vi "Mapping v10.6.3.2.vi"(5 "Simulate Spectra":bool, 7 "Simulate Drive":bool) -> ()   [LabVIEW 2010]
uses:
  TypeDefs/Mapping Spectra Params.ctl
  TypeDefs/Mapping Drive Params v10.6.0.ctl
  NPC3SG/TypeDefs/NPC3SG Set Positions.ctl
  NPC3SG/TypeDefs/NPC3SG Current Values.ctl
  iHR550/TypeDefs/iHR Current Values.ctl
  ITC503/TypeDefs/ITC503 Current Values.ctl
  TypeDefs/Mapping Input Parameters v10.6.2.ctl
  Symphony/TypeDefs/Symphony Area Format.ctl
  <vilib>/Utility/miscctls.llb/LVPointTypeDef.ctl
  Global Variables.vi
panel:
  in  "Measure Dummy 2":bool
  in  "Measure Dummy":bool
  in  "AutoSave Inc.":i16=20 caption="Auto Save (%)" min=10 max=160 step=1
  in  "Save Map":bool
  in  "Input Parameters":T1={"Drive Connection Port"="", "ITC503 Current Values"={"ITC503 Heater"=0.0, "ITC503 Temperature"=0.0, "ITC503 P"=0.0, "ITC503 I"=0.0, "ITC503 D"=0.0, "ITC503 Setpoint"=0.0, "ITC503 Gradient"=0.0, "ITC503 Heater Auto"=FALSE, "ITC503 PID Auto"=FALSE}, "Wavelengths (nm)"=[], "Drive Current Values"={"Drive X Position"=0.0, "Drive Y Position"=0.0, "Drive Z Position"=0.0}, "iHR Current Values"={"iHR 550 Front Entrance"=0.0, "iHR550 Side Exit"=0.0, "iHR550 Wavelength"=897.9988, "iHR550 Exit Mirror"=2, "iHR550 Grating"="1", "Grating Index"=1}, "Spectra Settings"={"Integration Time"=1.0, "Repetitions"=1, "Mapping Spectra"=TRUE}, "CCD3500 Temperature"=0.0, "Simulate Drive"=FALSE, "Simulate Spectra"=FALSE, "JYCCDLib.IJYCCDReqd"=refnum, "CCD Area"={"XStart"=1, "YStart"=1, "XStop"=2048, "YStop"=512, "XBin"=1, "YBin"=1}, "CCD Gain"=1, "CCD ADC"=0, "Drive Calibration"=path ""} {"CCD ADC" items=["20 kHz       ", " 1 MHz       ", " 1 MHz Ultra ", "500 kHz Wrap"]; "CCD Gain" items=["High Light", "Best Dynamic Range", "High Sensitivity"]; "ITC503 Current Values"."ITC503 Gradient" format="%.2f"; "ITC503 Current Values"."ITC503 Setpoint" min=-273.0 max=300000.0 step=0.0001 format="%.1f"; "ITC503 Current Values"."ITC503 I" format="%_1f"; "ITC503 Current Values"."ITC503 P" format="%_1f"; "ITC503 Current Values"."ITC503 Temperature" min=0.0 max=1645.0 step=1e-05 format="%.2f"; "ITC503 Current Values"."ITC503 Heater" min=0.0 max=100.0 step=0.01 scale=0.0..100.0; "Drive Current Values"."Drive Z Position" min=-273.0 max=300000.0 step=0.0001 format="%.3f"; "Drive Current Values"."Drive Y Position" min=-273.0 max=300000.0 step=0.0001 format="%.3f"; "Drive Current Values"."Drive X Position" min=-273.0 max=300000.0 step=0.0001 format="%.3f"; "iHR Current Values"."iHR550 Exit Mirror" items=["EntranceMirror", "ExitMirror", "Front", "Side"]; "Spectra Settings"."Repetitions" min=1 max=100 step=1; "Spectra Settings"."Integration Time" min=0.5 max=6000.0 step=1.0 format="%.1f"}
  out "JYCCDLib.IJYCCDReqd":refnum<k7>
  out "AutoClose":bool
  out "ITC503 Temperature":dbl caption="Sample (K)" min=10.0 max=160.0 step=0.1 format="%.3f"
  out "CCD3500 Temperature":dbl caption="CCD (°C)" min=10.0 max=160.0 step=0.1 format="%.1f"
  in  "CCD Current Rep.":string="0/0"
  in  "Pause":bool
  out "Current Position":T3 {"Drive Z Position" min=-273.0 max=300000.0 step=0.0001 format="%.3f"; "Drive Y Position" min=-273.0 max=300000.0 step=0.0001 format="%.3f"; "Drive X Position" min=-273.0 max=300000.0 step=0.0001 format="%.3f"}
  out "Target Position":T7={"Drive X Set"=10.0, "Drive Y Set"=10.0, "Drive Z Set"=10.0} {"Drive X Set" min=10.0 max=160.0 step=0.1 format="%.3f"; "Drive Z Set" min=10.0 max=160.0 step=0.1 format="%.3f"; "Drive Y Set" min=10.0 max=160.0 step=0.1 format="%.3f"}
  out "Progress":u8(slide) max=10 scale=0.0..100.0
  out "Objective Running":bool caption="Obj."
  out "CCD Running":bool caption="CCD"
  in  "Spectra Params":T5={"Integration Time"=10.0, "Repetitions"=10, "Mapping Spectra"=TRUE} {"Repetitions" min=1 max=100 step=1; "Integration Time" min=0.5 max=6000.0 step=1.0 format="%.1f"}
  in  "Drive Settings":refnum<visa-resource-name>
  in  "Z Position":dbl caption="Z (µm)" min=0.0 max=100.0 step=0.1 format="%.1f"
  in  "Mapping Params":T8={"X Start Position"=0.0, "X Stop Position"=10.0, "Y Start Position"=0.0, "Y Stop Position"=10.0, "Step Size"=1.0} {"Step Size" min=0.005 max=20.0 step=0.005 format="%.3f"; "Y Stop Position" min=0.0 max=140.0 step=0.005 format="%.3f"; "Y Start Position" min=0.0 max=140.0 step=0.005 format="%.3f"; "X Stop Position" min=0.0 max=140.0 step=0.005 format="%.3f"; "X Start Position" min=0.0 max=140.0 step=0.005 format="%.3f"}
  in  "Exit":bool
  out "Measuring":bool
  in  "Start":bool
  out "Filename":string
  out "Full Data":dbl[][](array[numeric])
  out "Live Data":dbl[][](array[numeric])
  in  "ITC503 Current Values":T2 {"ITC503 Gradient" format="%.2f"; "ITC503 Setpoint" min=-273.0 max=300000.0 step=0.0001 format="%.1f"; "ITC503 I" format="%_1f"; "ITC503 P" format="%_1f"; "ITC503 Temperature" min=0.0 max=1645.0 step=1e-05 format="%.2f"; "ITC503 Heater" min=0.0 max=100.0 step=0.01 scale=0.0..100.0}
  in  "iHR Current Values":T4={"iHR 550 Front Entrance"=0.0, "iHR550 Side Exit"=0.0, "iHR550 Wavelength"=897.9988, "iHR550 Exit Mirror"=2, "iHR550 Grating"="1", "Grating Index"=1} {"iHR550 Exit Mirror" items=["EntranceMirror", "ExitMirror", "Front", "Side"]}
  in  "Wavelengths (nm)":dbl[](array[numeric])
  # "Mapping"
  # "Status"
  # "Active"
  # "Target"
  # "Current"
  # "Spectral"
  # "Spectral / Video Mapping"
  # "Drive Settings"
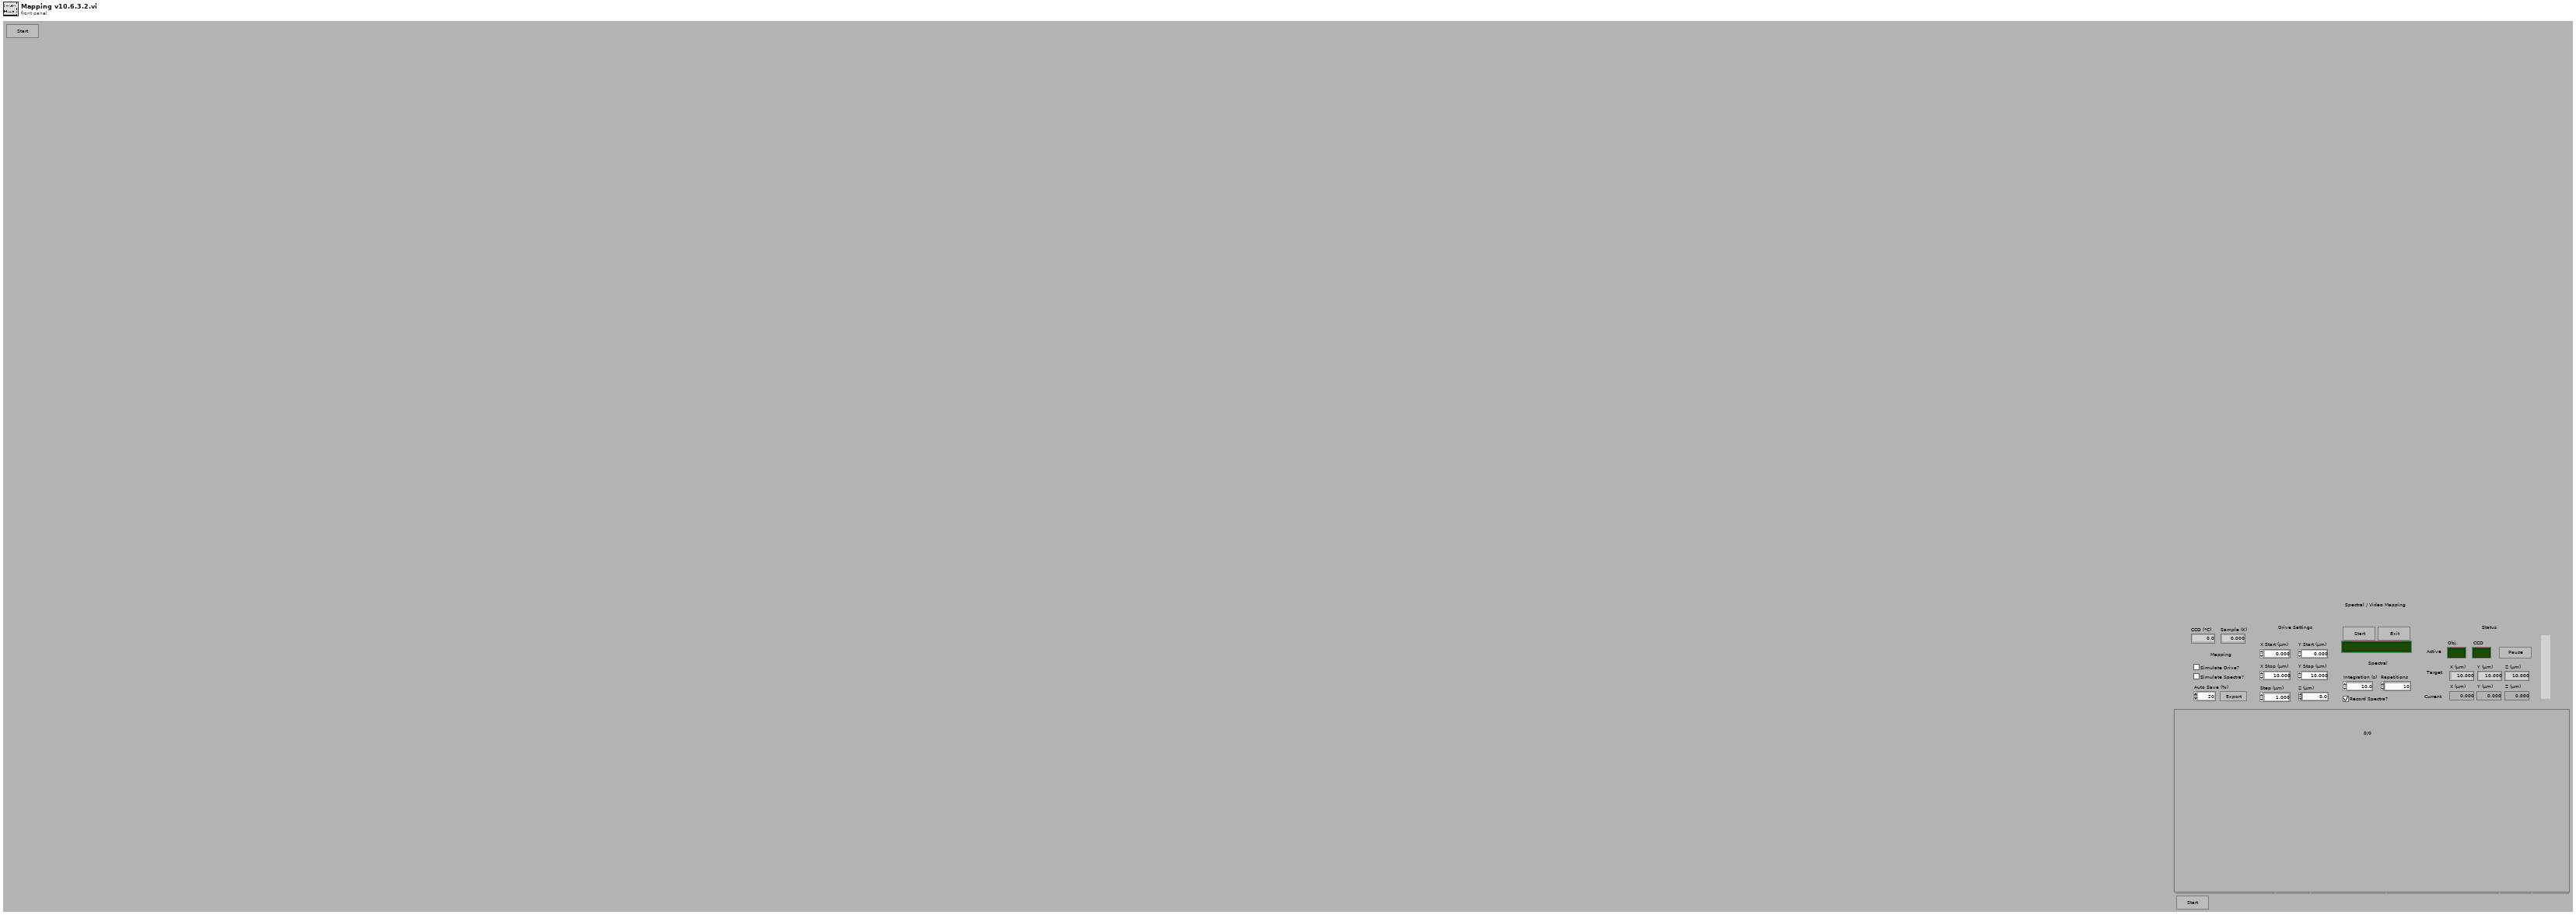
[diagram p1: front panel]
types:
  T1 = typedef "Mapping Input Parameters v10.6.2.ctl" = cluster{"Drive Connection Port":refnum<visa-resource-name>, "ITC503 Current Values":T2, "Wavelengths (nm)":dbl[], "Drive Current Values":T3, "iHR Current Values":T4, "Spectra Settings":T5, "CCD3500 Temperature":dbl, "Simulate Drive":bool, "Simulate Spectra":bool, "JYCCDLib.IJYCCDReqd":refnum<k7>, "CCD Area":T6, "CCD Gain":u16, "CCD ADC":u16, "Drive Calibration":path}
  T2 = typedef "ITC503 Current Values.ctl" = cluster{"ITC503 Heater":dbl, "ITC503 Temperature":dbl, "ITC503 P":dbl, "ITC503 I":dbl, "ITC503 D":dbl, "ITC503 Setpoint":dbl, "ITC503 Gradient":dbl, "ITC503 Heater Auto":bool, "ITC503 PID Auto":bool}
  T3 = typedef "NPC3SG Current Values.ctl" = cluster{"Drive X Position":dbl, "Drive Y Position":dbl, "Drive Z Position":dbl}
  T4 = typedef "iHR Current Values.ctl" = cluster{"iHR 550 Front Entrance":dbl, "iHR550 Side Exit":dbl, "iHR550 Wavelength":dbl, "iHR550 Exit Mirror":i32, "iHR550 Grating":string, "Grating Index":i32}
  T5 = typedef "Mapping Spectra Params.ctl" = cluster{"Integration Time":dbl, "Repetitions":u16, "Mapping Spectra":bool}
  T6 = typedef "Symphony Area Format.ctl" = cluster{"XStart":i32, "YStart":i32, "XStop":i32, "YStop":i32, "XBin":i32, "YBin":i32}
  T7 = typedef "NPC3SG Set Positions.ctl" = cluster{"Drive X Set":dbl, "Drive Y Set":dbl, "Drive Z Set":dbl}
  T8 = typedef "Mapping Drive Params v10.6.0.ctl" = cluster{"X Start Position":dbl, "X Stop Position":dbl, "Y Start Position":dbl, "Y Stop Position":dbl, "Step Size":dbl}
  T9 = typedef "LVPointTypeDef.ctl" = cluster{"Horizontal":i16, "Vertical":i16}
  T10 = cluster{"Intensities":dbl[], "Wavelengths":dbl[]}[]
  T11 = cluster{"Intensities":dbl[], "Wavelengths":dbl[]}
  T12 = enum32{"invalid app kind", "Development System", "Run Time System", "Student Edition", "Embedded LabVIEW", "Evaluation", "Custom"}
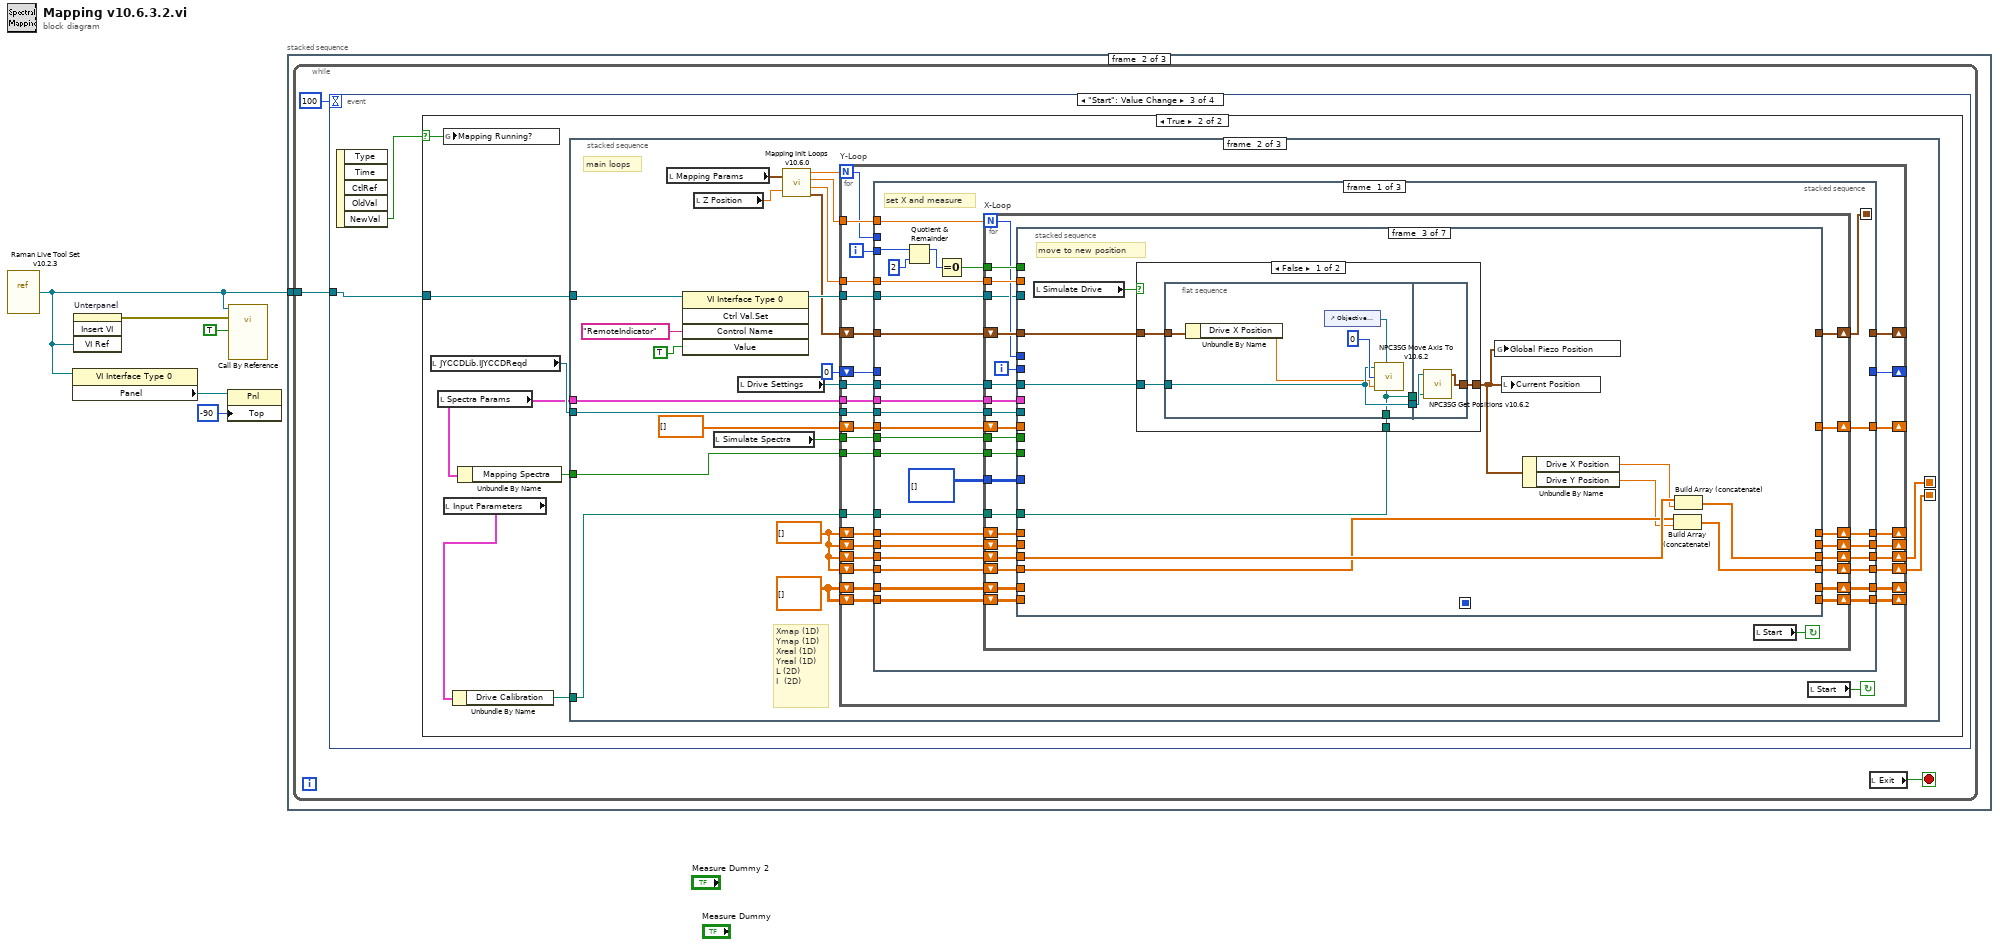
[diagram p0: block diagram]
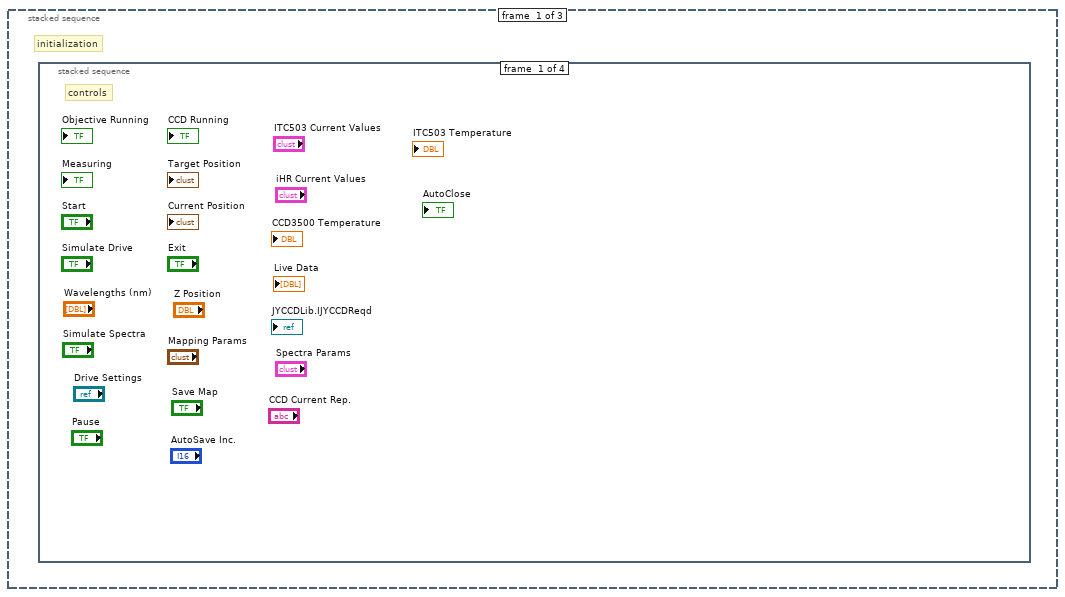
[diagram p2: hidden frame]
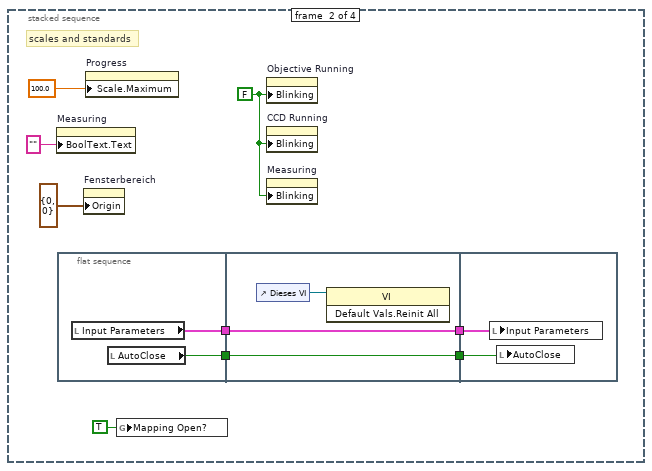
[diagram p3: hidden frame]
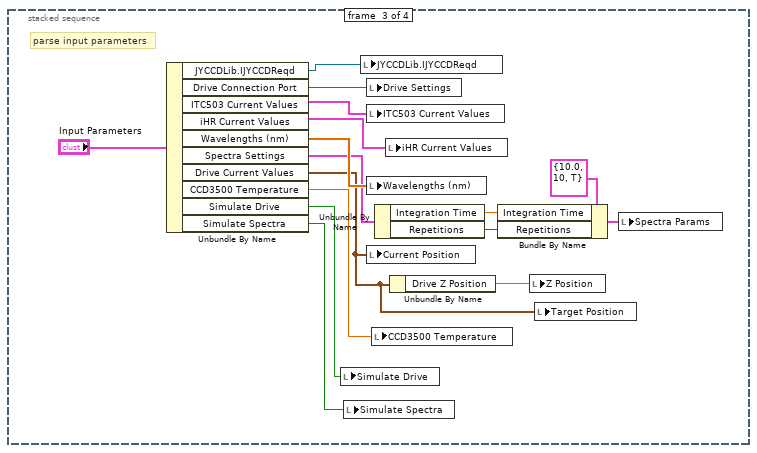
[diagram p4: hidden frame]
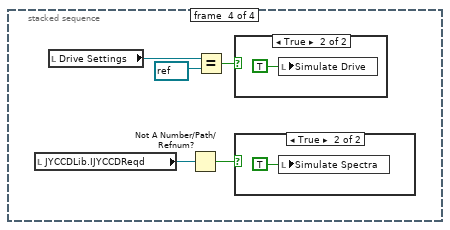
[diagram p5: hidden frame]
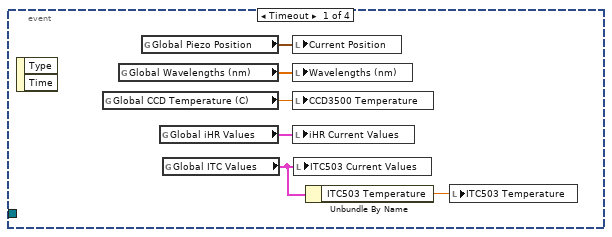
[diagram p8: hidden frame]
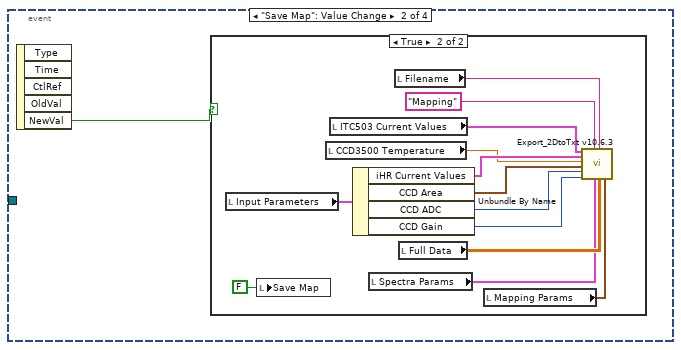
[diagram p9: hidden frame]
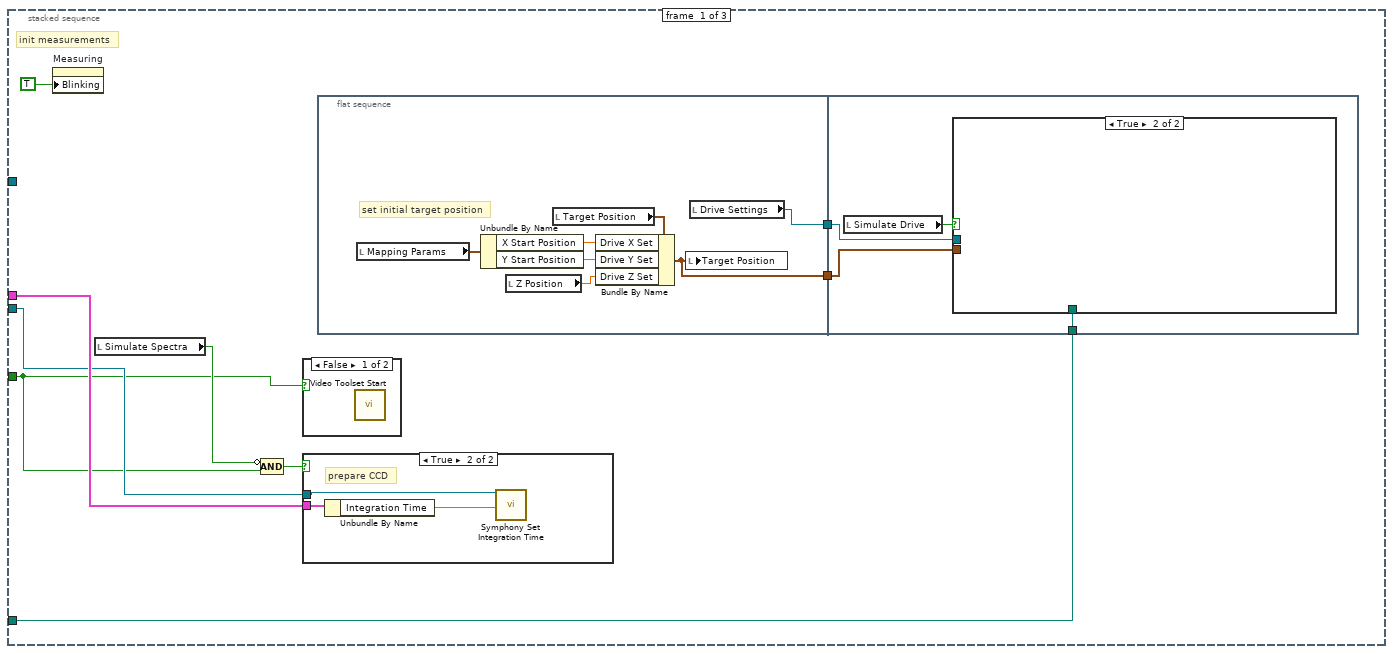
[diagram p12: hidden frame]
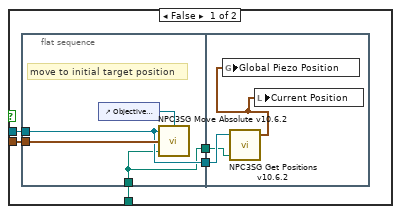
[diagram p15: hidden frame]
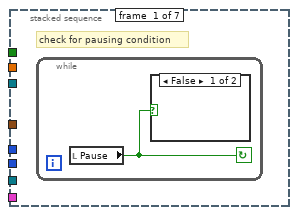
[diagram p16: hidden frame]
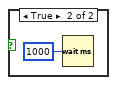
[diagram p17: hidden frame]
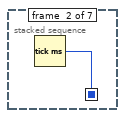
[diagram p18: hidden frame]
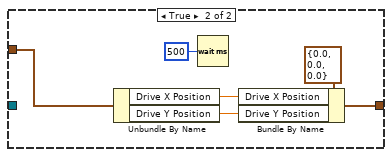
[diagram p19: hidden frame]
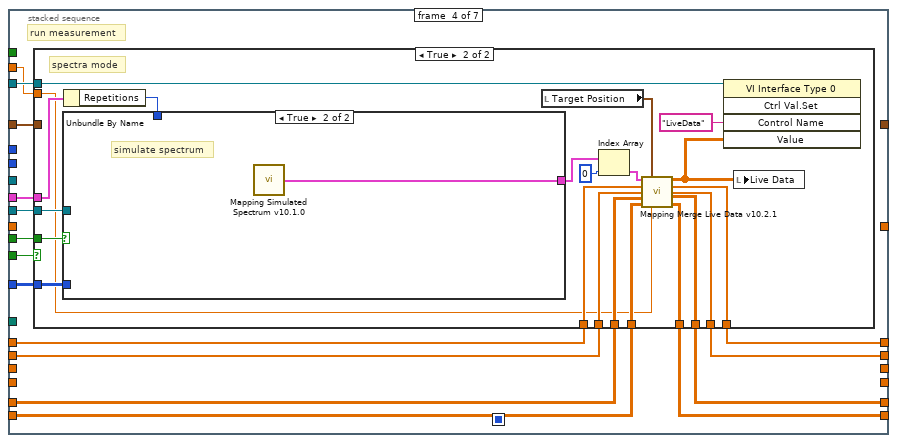
[diagram p20: hidden frame]
diagram:
  n1 = vi-ref "Raman Live Tool Set v10.2.3.vi"() -> (w3:refnum<vi>)
  n2 = property class="VI Interface Type 0"(reference=w3) -> ("Panel"=w2:refnum<vi>)  [unwired: 1 in, 2 out]
  n3 = invoke on="Unterpanel" class="Unterpanel" method="Insert VI"("VI Ref"=w3) -> (error out=w5:errorcluster)  [unwired: 3 in, 3 out]
  n4 = property class="Pnl"(reference=w2, "Top"=-90 ("Position:Oben")) -> ()  [unwired: 1 in, 2 out]
  n5 = call-by-ref "?"(reference=w3, error in=w5, "RemoteIndicator"=TRUE) -> ()  [unwired: 3 in, 2 out]
  n6 = stacked-sequence {
    tunnel: w3 -> [_ w45 w474]
    frame #0 {
      # "initialization"
      n7 = stacked-sequence {
        frame #0 {
          # "controls"
        }
        frame #1 {
          w12 = FALSE ("Blinkend")
          # "scales and standards"
          n8 = property on="Measuring" class="Bool (strict)"("BoolText.Text"="" ("Boolescher Text.Text")) -> ()  [unwired: 2 in, 2 out]
          n9 = flat-sequence {
            tunnel: [w16] -> w9
            tunnel: [w15] -> w6
            tunnel: [w18] -> w10
            tunnel: w9 -> [w18]
            tunnel: [w17] -> w7
            tunnel: w6 -> [w17]
            tunnel: w10 -> [w21]
            tunnel: w7 -> [w20]
            frame #0 {
              n10 = local read "Input Parameters"() -> (w16:T1)
              n11 = local read "AutoClose"() -> (w15:bool)
            }
            frame #1 {
              n12 = control-ref of="Dieses VI"() -> (w19:refnum<vi>)
              n13 = invoke class="VI" method="Default Vals.Reinit All"(reference=w19) -> ()  [unwired: 2 in, 3 out]
            }
            frame #2 {
              n14 = local write "Input Parameters"(w21) -> ()
              n15 = local write "AutoClose"(w20) -> ()
            }
          }
          n16 = property on="Fensterbereich" class="Pane"("Origin"=T9 {"Horizontal"=0, "Vertical"=0}) -> ()  [unwired: 2 in, 2 out]
          n17 = property on="Progress" class="Slide (strict)"("Scale.Maximum"=100.0 ("Skalierung.Bereich:Maximum")) -> ()  [unwired: 2 in, 2 out]
          n18 = global write "Global Variables.vi" "Mapping Open?"(TRUE ("Mapping Open?")) -> ()
          n19 = property on="Objective Running" class="Bool (strict)"("Blinking"=w12) -> ()  [unwired: 2 in, 2 out]
          n20 = property on="CCD Running" class="Bool (strict)"("Blinking"=w12) -> ()  [unwired: 2 in, 2 out]
          n21 = property on="Measuring" class="Bool (strict)"("Blinking"=w12) -> ()  [unwired: 2 in, 2 out]
        }
        frame #2 {
          # "parse input parameters"
          n22 = Unbundle By Name("Input Parameters") -> ("JYCCDLib.IJYCCDReqd"=w25:refnum<k7>, "Drive Connection Port"=w22:refnum<visa-resource-name>, "ITC503 Current Values"=w37:T2, "iHR Current Values"=w28:T4, "Wavelengths (nm)"=w36:dbl[], "Spectra Settings"=w34:T5, "Drive Current Values"=w23:T3, "CCD3500 Temperature"=w29:dbl, "Simulate Drive"=w27:bool, "Simulate Spectra"=w26:bool)
          n23 = local write "Simulate Drive"(w27) -> ()
          n24 = local write "Simulate Spectra"(w26) -> ()
          n25 = local write "JYCCDLib.IJYCCDReqd"(w25) -> ()
          n26 = local write "Drive Settings"(w22) -> ()
          n27 = local write "ITC503 Current Values"(w37) -> ()
          n28 = local write "Wavelengths (nm)"(w36) -> ()
          n29 = local write "Current Position"(w23) -> ()
          n30 = local write "CCD3500 Temperature"(w29) -> ()
          n31 = Unbundle By Name(w34) -> ("Integration Time"=w32:dbl, "Repetitions"=w31:u16)
          n32 = local write "iHR Current Values"(w28) -> ()
          n33 = Unbundle By Name(w23) -> ("Drive Z Position"=w35:dbl)
          n34 = Bundle By Name(cluster=T5 {"Integration Time"=10.0, "Repetitions"=10, "Mapping Spectra"=TRUE} ("Mapping Spectra Settings"), "Integration Time"=w32, "Repetitions"=w31) -> (w30:T5)
          n35 = local write "Z Position"(w35) -> ()
          n36 = local write "Target Position"(w23) -> ()
          n37 = local write "Spectra Params"(w30) -> ()
        }
        frame #3 {
          n38 = local read "JYCCDLib.IJYCCDReqd"() -> (w39:refnum<k7>)
          n39 = local read "Drive Settings"() -> (w40:refnum<visa-resource-name>)
          n40 = Not A Number/Path/Refnum?(number/path/refnum=w39) -> (NaN/Path/Refnum?=w38:bool)
          n41 = Equal?(x=w40, y=refnum<visa-resource-name> refnum ("Drive Settings")) -> (x = y?=w41:bool)
          n42 = case shown="True" w41 {
            frame False {
            }
            frame True {
              n43 = local write "Simulate Drive"(TRUE ("Simulate Drive")) -> ()
            }
          }
          n44 = case shown="True" w38 {
            frame False {
            }
            frame True {
              n45 = local write "Simulate Spectra"(TRUE ("Simulate Drive")) -> ()
            }
          }
        }
      }
    }
    frame #1 {
      n46 = while {
        tunnel: w45 -> [w48]
        stop <- w47 stop-if-true
        n47 = event shown="[2] \"Start\": Value Change" {
          selector: _ -> [_ _ _ _]
          dyn-events: _ -> [_ _ _ _]
          timeout: 100 -> [_ _ _ _]
          tunnel: w48 -> [_ _ w69 _]
          event Timeout {
            n48 = event-data() -> ()  [unwired: 1 in, 2 out]
            n49 = global read "Global Variables.vi" "Global CCD Temperature (C)"() -> (w54:dbl)
            n50 = global read "Global Variables.vi" "Global Wavelengths (nm)"() -> (w52:dbl[])
            n51 = global read "Global Variables.vi" "Global Piezo Position"() -> (w53:T3)
            n52 = global read "Global Variables.vi" "Global iHR Values"() -> (w51:T4)
            n53 = global read "Global Variables.vi" "Global ITC Values"() -> (w50:T2)
            n54 = local write "Current Position"(w53) -> ()
            n55 = local write "Wavelengths (nm)"(w52) -> ()
            n56 = local write "CCD3500 Temperature"(w54) -> ()
            n57 = local write "iHR Current Values"(w51) -> ()
            n58 = local write "ITC503 Current Values"(w50) -> ()
            n59 = Unbundle By Name(w50) -> ("ITC503 Temperature"=w49:dbl)
            n60 = local write "ITC503 Temperature"(w49) -> ()
          }
          event "Save Map": Value Change {
            n61 = event-data() -> ("NewVal"=w55:bool)  [unwired: 1 in, 4 out]
            n62 = case shown="True" w55 {
              frame False {
              }
              frame True {
                n63 = local read "Input Parameters"() -> (w64:T1)
                n64 = local write "Save Map"(FALSE ("Save Map")) -> ()
                n65 = local read "CCD3500 Temperature"() -> (w58:dbl)
                n66 = local read "ITC503 Current Values"() -> (w61:T2)
                n67 = Unbundle By Name(w64) -> ("iHR Current Values"=w59:T4, "CCD Area"=w60:T6, "CCD ADC"=w63:u16, "CCD Gain"=w62:u16)
                n68 = local read "Spectra Params"() -> (w57:T5)
                n69 = local read "Filename"() -> (w67:string)
                n70 = local read "Full Data"() -> (w65:dbl[][])
                n71 = local read "Mapping Params"() -> (w56:T8)
                n72 = call "Export_2DtoTxt v10.6.3.vi"("ITC503 Current Values"=w61, "iHR Current Values"=w59, "CCD Temperature"=w58, "CCD Area"=w60, "CCD ADC"=w63, "CCD Gain"=w62, "Export Type"="Mapping", "Spectra Settings"=w57, "Filename"=w67, "Data (2D)"=w65, "Mapping Parameters"=w56) -> ()  [unwired: 8 in, 1 out]
              }
            }
          }
          event "Start": Value Change {
            n73 = event-data() -> ("NewVal"=w70:bool)  [unwired: 1 in, 4 out]
            n74 = case shown="True" w70 {
              selector: w70 -> [_ w74]
              tunnel: w69 -> [_ w77]
              frame False {
              }
              frame True {
                n75 = local read "JYCCDLib.IJYCCDReqd"() -> (w76:refnum<k7>)
                n76 = local read "Spectra Params"() -> (w75:T5)
                n77 = global write "Global Variables.vi" "Mapping Running?"(w74) -> ()
                n78 = local read "Input Parameters"() -> (w72:T1)
                n79 = Unbundle By Name(w72) -> ("Drive Calibration"=w71:path)
                n80 = Unbundle By Name(w75) -> ("Mapping Spectra"=w73:bool)
                n81 = stacked-sequence {
                  seq-local: [_ w115 _] -> [_ _ w449]
                  seq-local: [_ w116 _] -> [_ _ w448]
                  tunnel: w77 -> [_ w126 _]
                  tunnel: w73 -> [w79 w125 w450]
                  tunnel: w75 -> [w81 w123 _]
                  tunnel: w76 -> [w80 w122 _]
                  tunnel: w71 -> [w78 w114 _]
                  frame #0 {
                    # "init measurements"
                    n82 = property on="Measuring" class="Bool (strict)"("Blinking"=TRUE ("Blinkend")) -> ()  [unwired: 2 in, 2 out]
                    n83 = local read "Simulate Spectra"() -> (w83:bool)
                    n84 = Compound Arithmetic op=AND(invert w83, w79) -> (w82:bool)
                    n85 = case shown="False" w79 {
                      frame False {
                        n86 = call "Video Toolset Start.vi"() -> ()  [unwired: 3 in]
                      }
                      frame True {
                      }
                    }
                    n87 = case shown="True" w82 {
                      tunnel: w80 -> [_ w89]
                      tunnel: w81 -> [_ w88]
                      frame False {
                      }
                      frame True {
                        # "prepare CCD"
                        n88 = Unbundle By Name(w88) -> ("Integration Time"=w87:dbl)
                        n89 = call "Symphony Set Integration Time.vi"("JYCCDLib.IJYCCDReqd"=w89, "Integration (s)"=w87) -> ()  [unwired: 13 in, 1 out]
                      }
                    }
                    n90 = flat-sequence {
                      tunnel: [w91] -> w85
                      tunnel: [w90] -> w84
                      tunnel: w85 -> [w98]
                      tunnel: w84 -> [w99]
                      tunnel: w78 -> [w97]
                      frame #0 {
                        # "set initial target position"
                        n91 = local read "Mapping Params"() -> (w96:T8)
                        n92 = Unbundle By Name(w96) -> ("X Start Position"=w94:dbl, "Y Start Position"=w93:dbl)
                        n93 = local read "Z Position"() -> (w92:dbl)
                        n94 = local read "Target Position"() -> (w95:T7)
                        n95 = Bundle By Name(cluster=w95, "Drive X Set"=w94, "Drive Y Set"=w93, "Drive Z Set"=w92) -> (w91:T7)
                        n96 = local write "Target Position"(w91) -> ()
                        n97 = local read "Drive Settings"() -> (w90:refnum<visa-resource-name>)
                      }
                      frame #1 {
                        n98 = local read "Simulate Drive"() -> (w100:bool)
                        n99 = case shown="True" w100 {
                          tunnel: w99 -> [w105 _]
                          tunnel: w98 -> [w103 _]
                          tunnel: w97 -> [w102 _]
                          frame False {
                            n100 = flat-sequence {
                              tunnel: w105 -> [w107]
                              tunnel: [w107] -> w104
                              tunnel: w103 -> [w108]
                              tunnel: w102 -> [w106]
                              tunnel: [w106] -> w101
                              tunnel: w104 -> [w111]
                              tunnel: w101 -> [w110]
                              frame #0 {
                                # "move to initial target position"
                                n101 = control-ref of="Objective Running"() -> (w109:refnum<vi>)
                                n102 = call "NPC3SG Move Absolute v10.6.2.vi"("Running"=w109, "Calibration File"=w106, "Drive New Abs. Positions"=w108, "Drive Visa Name"=w107) -> ()  [unwired: 1 in]
                              }
                              frame #1 {
                                n103 = call "NPC3SG Get Positions v10.6.2.vi"("Drive Visa Name"=w111, "Calibration File"=w110) -> ("Drive Current Values"=w112:T3)  [unwired: 5 in]
                                n104 = global write "Global Variables.vi" "Global Piezo Position"(w112) -> ()
                                n105 = local write "Current Position"(w112) -> ()
                              }
                            }
                          }
                          frame True {
                          }
                        }
                      }
                    }
                  }
                  frame #1 {
                    w134 = dbl[][] []
                    w117 = dbl[] []
                    # "main loops"
                    # "Xmap (1D)\nYmap (1D)\nXreal (1D)\nYreal (1D)\nL (2D)\nI  (2D)"
                    n106 = local read "Mapping Params"() -> (w120:T8)
                    n107 = invoke class="VI Interface Type 0" method="Ctrl Val.Set"(reference=w126, "Control Name"="RemoteIndicator" ("Elementname"), "Value"=TRUE) -> (reference out=w128:refnum<vi>)  [unwired: 2 in, 4 out]
                    n108 = local read "Z Position"() -> (w119:dbl)
                    n109 = local read "Simulate Spectra"() -> (w118:bool)
                    n110 = local read "Drive Settings"() -> (w121:refnum<visa-resource-name>)
                    n111 = call "Mapping Init Loops v10.6.0.vi"("Z Position"=w119, "Mapping Params"=w120) -> ("Start Positions"=w127:T3, "Step Size"=w129:dbl, "X Steps"=w130:dbl, "Y Steps"=w131:dbl)
                    n112 = for "Y-Loop" {
                      N: w131 -> [w150]
                      tunnel: w130 -> [w163]
                      tunnel: w129 -> [w162]
                      shift-right: [w148] -> _
                      shift-left: w127 -> [w149]
                      shift-right: [w154] -> _
                      shift-left: w134 -> [w158]
                      shift-right: [w155] -> _
                      shift-left: w134 -> [w159]
                      shift-right: [w157] -> _
                      shift-left: w117 -> [w161]
                      shift-right: [w156] -> _
                      shift-left: w117 -> [w160]
                      tunnel: w128 -> [w152]
                      tunnel: w118 -> [w151]
                      tunnel: w121 -> [w147]
                      tunnel: w125 -> [w146]
                      tunnel: w123 -> [w145]
                      shift-right: [w143] -> _
                      shift-left: dbl[] [] -> [w144]
                      tunnel: w122 -> [w142]
                      shift-right: [w139] -> w116
                      shift-left: w117 -> [w140]
                      shift-right: [w138] -> w115
                      shift-left: w117 -> [w141]
                      tunnel: w114 -> [w137]
                      shift-right: [w136] -> _
                      shift-left: i16 0 ("Progress") -> [w135]
                      i -> [w153]
                      stop <- w164 continue-if-true
                      n113 = stacked-sequence {
                        seq-local: [w179 _ _] -> [_ _ w419]
                        tunnel: w163 -> [w194 _ _]
                        tunnel: w162 -> [w193 _ w420]
                        tunnel: w161 -> [w192 _ _]
                        tunnel: w160 -> [w191 _ _]
                        tunnel: w159 -> [w190 _ _]
                        tunnel: w158 -> [w166 _ _]
                        tunnel: [w189 _ _] -> w157
                        tunnel: [w188 _ _] -> w156
                        tunnel: [w187 _ _] -> w155
                        tunnel: [w186 _ _] -> w154
                        tunnel: w153 -> [w183 _ w423]
                        tunnel: w152 -> [w181 _ _]
                        tunnel: w151 -> [w180 _ _]
                        tunnel: w150 -> [_ _ w421]
                        tunnel: w149 -> [w178 _ _]
                        tunnel: [_ _ w417] -> w148
                        tunnel: w147 -> [w177 _ w418]
                        tunnel: w146 -> [w176 _ _]
                        tunnel: w145 -> [w175 _ _]
                        tunnel: w144 -> [w174 _ _]
                        tunnel: [w173 _ _] -> w143
                        tunnel: w142 -> [w172 _ _]
                        tunnel: w141 -> [w170 w385 _]
                        tunnel: w140 -> [w169 w384 _]
                        tunnel: [w168 _ _] -> w139
                        tunnel: [w167 _ _] -> w138
                        tunnel: w137 -> [w165 _ w411]
                        tunnel: [_ w383 _] -> w136
                        tunnel: w135 -> [_ w382 _]
                        frame #0 {
                          # "set X and measure"
                          n114 = Quotient & Remainder(x=w183, y=2) -> (x-y*floor(x/y)=w184:i32)  [unwired: 1 out]
                          n115 = Equal To 0?(x=w184) -> (x = 0?=w182:bool)
                          n116 = for "X-Loop" {
                            N: w194 -> [w209]
                            tunnel: w193 -> [w221]
                            shift-right: [w220] -> w179
                            shift-left: w178 -> [w222]
                            shift-right: [w215] -> w189
                            shift-left: w192 -> [w219]
                            shift-right: [w214] -> w188
                            shift-left: w191 -> [w218]
                            shift-right: [w212] -> w187
                            shift-left: w190 -> [w217]
                            shift-right: [w213] -> w186
                            shift-left: w166 -> [w216]
                            tunnel: w182 -> [w211]
                            tunnel: w181 -> [w208]
                            tunnel: w180 -> [w207]
                            tunnel: w177 -> [w206]
                            tunnel: w176 -> [w205]
                            tunnel: w175 -> [w204]
                            shift-right: [w203] -> w173
                            shift-left: w174 -> [w202]
                            tunnel: w172 -> [w201]
                            tunnel: u16[][] [] -> [w200]
                            shift-right: [w196] -> w167
                            shift-left: w170 -> [w199]
                            shift-right: [w197] -> w168
                            shift-left: w169 -> [w198]
                            tunnel: w165 -> [w195]
                            i -> [w210]
                            stop <- w223 continue-if-true
                            n117 = stacked-sequence {
                              seq-local: [_ w226 _ _ _ _ _] -> [_ _ _ _ _ w361 _]
                              tunnel: w222 -> [_ _ w237 w274 w338 _ _]
                              tunnel: w221 -> [_ _ _ w259 w336 _ _]
                              tunnel: [_ _ _ _ w335 _ _] -> w220
                              tunnel: w219 -> [_ _ _ w273 _ _ _]
                              tunnel: w218 -> [_ _ _ w272 _ _ _]
                              tunnel: w217 -> [_ _ _ w270 _ _ _]
                              tunnel: w216 -> [_ _ _ w271 _ _ w370]
                              tunnel: [_ _ _ w269 _ _ _] -> w215
                              tunnel: [_ _ _ w268 _ _ _] -> w214
                              tunnel: [_ _ _ w267 _ _ _] -> w213
                              tunnel: [_ _ _ w266 _ _ _] -> w212
                              tunnel: w211 -> [_ _ _ _ w337 _ _]
                              tunnel: w210 -> [_ _ _ _ w341 _ _]
                              tunnel: w209 -> [_ _ _ _ w339 _ _]
                              tunnel: w208 -> [_ _ _ w265 _ _ _]
                              tunnel: w207 -> [_ _ _ w264 _ _ _]
                              tunnel: w206 -> [_ _ w235 _ _ _ _]
                              tunnel: w205 -> [_ _ _ w263 _ _ _]
                              tunnel: w204 -> [_ _ _ w261 _ _ w372]
                              tunnel: [_ _ _ _ _ w358 _] -> w203
                              tunnel: w202 -> [_ _ _ _ _ w360 w371]
                              tunnel: w201 -> [_ _ _ w262 _ _ _]
                              tunnel: w200 -> [_ _ _ w260 _ _ _]
                              tunnel: w199 -> [_ _ w234 _ _ _ _]
                              tunnel: w198 -> [_ _ w233 _ _ _ _]
                              tunnel: [_ _ w230 _ _ _ _] -> w197
                              tunnel: [_ _ w229 _ _ _ _] -> w196
                              tunnel: w195 -> [_ _ w227 _ _ _ _]
                              frame #0 {
                                # "check for pausing condition"
                                n118 = while {
                                stop <- w224 continue-if-true
                                n119 = local read "Pause"() -> (w224:bool)
                                n120 = case shown="False" w224 {
                                frame False {
                                }
                                frame True {
                                n121 = Wait (ms)(milliseconds to wait=u32 1000) -> ()  [unwired: 1 out]
                                }
                                }
                                }
                              }
                              frame #1 {
                                n122 = Tick Count (ms)() -> (millisecond timer value=w226:u32)
                              }
                              frame #2 {
                                # "move to new position"
                                n123 = local read "Simulate Drive"() -> (w236:bool)
                                n124 = case shown="False" w236 {
                                tunnel: w237 -> [w243 w257]
                                tunnel: w235 -> [w242 _]
                                tunnel: [w240 w253] -> w228
                                tunnel: w227 -> [w239 _]
                                frame False {
                                n125 = flat-sequence {
                                tunnel: w243 -> [w246]
                                tunnel: w242 -> [w247]
                                tunnel: [w247] -> w241
                                tunnel: w239 -> [w244]
                                tunnel: [w244] -> w238
                                tunnel: w241 -> [w252]
                                tunnel: [w251] -> w240
                                tunnel: w238 -> [w250]
                                frame #0 {
                                n126 = Unbundle By Name(w246) -> ("Drive X Position"=w245:dbl)
                                n127 = control-ref of="Objective Running"() -> (w248:refnum<vi>)
                                n128 = call "NPC3SG Move Axis To v10.6.2.vi"("Drive Visa Name"=w247, "Running"=w248, "Axis"=0, "Drive Set"=w245, "Calibration File"=w244) -> ()  [unwired: 2 in, 1 out]
                                }
                                frame #1 {
                                n129 = call "NPC3SG Get Positions v10.6.2.vi"("Drive Visa Name"=w252, "Calibration File"=w250) -> ("Drive Current Values"=w251:T3)  [unwired: 5 in]
                                }
                                }
                                }
                                frame True {
                                n130 = Unbundle By Name(w257) -> ("Drive X Position"=w258:dbl, "Drive Y Position"=w255:dbl)
                                n131 = Wait (ms)(milliseconds to wait=u32 500 ("Zu wartende ms")) -> ()  [unwired: 1 out]
                                n132 = Bundle By Name(cluster=T3 {"Drive X Position"=0.0, "Drive Y Position"=0.0, "Drive Z Position"=0.0} ("Drive Current Values"), "Drive X Position"=w258, "Drive Y Position"=w255) -> (w253:T3)
                                }
                                }
                                n133 = global write "Global Variables.vi" "Global Piezo Position"(w228) -> ()
                                n134 = local write "Current Position"(w228) -> ()
                                n135 = Unbundle By Name(w228) -> ("Drive X Position"=w232:dbl, "Drive Y Position"=w231:dbl)
                                n136 = Build Array (concatenate)(w233, w231) -> (w230:dbl[])
                                n137 = Build Array (concatenate)(w234, w232) -> (w229:dbl[])
                              }
                              frame #3 {
                                # "run measurement"
                                n138 = case shown="True" w263 {
                                tunnel: w274 -> [_ _]
                                tunnel: w273 -> [w281 w302]
                                tunnel: w272 -> [w280 w301]
                                tunnel: w271 -> [w283 w299]
                                tunnel: w270 -> [w284 w300]
                                tunnel: [w278 w296] -> w269
                                tunnel: [w279 w295] -> w268
                                tunnel: [w283 w298] -> w267
                                tunnel: [w284 w297] -> w266
                                tunnel: w265 -> [_ w304]
                                tunnel: w264 -> [_ w303]
                                tunnel: w262 -> [_ w292]
                                tunnel: w261 -> [_ w291]
                                tunnel: w260 -> [_ w289]
                                tunnel: w259 -> [_ w285]
                                frame False {
                                # "video mode (take snapshot)"
                                n139 = local read "Current Position"() -> (w282:T3)
                                n140 = Unbundle By Name(w282) -> ("Drive X Position"=w277:dbl, "Drive Y Position"=w276:dbl)
                                n141 = call "Video Toolset Snapshot.vi"() -> ()  [unwired: 12 in]
                                n142 = Build Array (concatenate)(w281, w277) -> (w278:dbl[])
                                n143 = Build Array (concatenate)(w280, w276) -> (w279:dbl[])
                                n144 = Build Array(w278, w279) -> (w275:dbl[][])
                                n145 = local write "Live Data"(w275) -> ()
                                }
                                frame True {
                                # "spectra mode"
                                n146 = Unbundle By Name(w291) -> ("Repetitions"=w290:u16)
                                n147 = case shown="True" w303 {
                                tunnel: [w308 w330] -> w288
                                tunnel: w292 -> [w309 _]
                                tunnel: w290 -> [w307 _]
                                tunnel: w289 -> [w306 _]
                                frame False {
                                n148 = for {
                                N: w307 -> [w316]
                                shift-right: [w327] -> _
                                shift-left: w306 -> [w328]
                                tunnel: [w325] -> w308
                                tunnel: w309 -> [w314]
                                i -> [w329]
                                stop <- w323 continue-if-true
                                n149 = Number To Decimal String(number=w316) -> (decimal integer string=w319:string)  [unwired: 1 in]
                                n150 = control-ref of="CCD Running"() -> (w322:refnum<vi>)
                                n151 = control-ref of="Start"() -> (w321:refnum<vi>)
                                n152 = call "Symphony Acquire Spectrum.vi"("Acquire"=w321, "Running"=w322, "ShutterOpen"=TRUE, "JYCCDLib.IJYCCDReqd"=w314) -> ("Raw Data"=w311:i32[][])  [unwired: 6 in, 1 out]
                                n153 = Index Array(array=w311, index (row)=0) -> (element=w310:i32[])  [unwired: 1 in]
                                n154 = local read "Wavelengths (nm)"() -> (w324:dbl[])
                                n155 = Increment(x=w329) -> (x+1=w315:i32)
                                n156 = Number To Decimal String(number=w315) -> (decimal integer string=w318:string)  [unwired: 1 in]
                                n157 = Concatenate Strings(w318, "/" ("string"), w319) -> (w317:string)
                                n158 = local write "CCD Current Rep."(w317) -> ()
                                n159 = Build Array (concatenate)(w310, w328) -> (w327:i32[][])
                                n160 = call "Symphony Average Spectra.vi"("Repetitions"=w315, "Raw Spectra"=w327) -> ("Raw Spectrum"=w326:dbl[])
                                n161 = local read "Start"() -> (w323:bool)
                                n162 = call "Spectrum Merge Wavelengths v10.5.0.vi"("Wavelengths (nm)"=w324, "Raw Spectrum"=w326) -> ("Spectrum-Cluster"=w325:T10)  [unwired: 1 out]
                                }
                                }
                                frame True {
                                # "simulate spectrum"
                                n163 = call "Mapping Simulated Spectrum v10.1.0.vi"() -> ("Simulated Spectrum"=w330:cluster{i32[], dbl[]}[])
                                }
                                }
                                n164 = local read "Target Position"() -> (w294:T7)
                                n165 = Index Array(array=w288, index=0 ("Index")) -> (element=w287:T11)
                                n166 = call "Mapping Merge Live Data v10.2.1.vi"("New Spectrum"=w287, "Target Position"=w294, "X in (1D)"=w302, "Y in (1D)"=w301, "L in (2D)"=w300, "I in (2D)"=w299, "Step Size"=w285) -> ("Live Data"=w293:dbl[][], "X out (1D)"=w296:dbl[], "Y out (1D)"=w295:dbl[], "L out (2D)"=w297:dbl[][], "I out (2D)"=w298:dbl[][])  [unwired: 4 in]
                                n167 = invoke class="VI Interface Type 0" method="Ctrl Val.Set"(reference=w304, "Control Name"="LiveData" ("Elementname"), "Value"=w293) -> ()  [unwired: 2 in, 5 out]
                                n168 = local write "Live Data"(w293) -> ()
                                }
                                }
                              }
                              frame #4 {
                                # "set new X"
                                n169 = Increment(x=w341) -> (x+1=w340:i32)
                                n170 = local read "Start"() -> (w334:bool)
                                n171 = Equal?(x=w339, y=w340) -> (x = y?=w331:bool)
                                n172 = Not(x=w334) -> (.not. x?=w333:bool)
                                n173 = Or(x=w331, y=w333) -> (x .or. y?=w332:bool)
                                n174 = case shown="False" w332 {
                                tunnel: w338 -> [w349 w357]
                                tunnel: [w348 w357] -> w335
                                tunnel: w337 -> [w347 _]
                                tunnel: w336 -> [w342 _]
                                frame False {
                                n175 = Unbundle By Name(w349) -> ("Drive X Position"=w350:dbl)
                                n176 = case shown="False" w347 {
                                tunnel: w350 -> [w353 w355]
                                tunnel: [w352 w356] -> w343
                                tunnel: w342 -> [w351 w354]
                                frame False {
                                n177 = Subtract(x=w353, y=w351) -> (x-y=w352:dbl)
                                }
                                frame True {
                                n178 = Add(x=w355, y=w354) -> (x+y=w356:dbl)
                                }
                                }
                                n179 = Divide(x=w343, y=w342) -> (x/y=w346:dbl)
                                n180 = Round To Nearest(number=w346) -> (nearest integer value=w345:dbl)
                                n181 = Multiply(x=w345, y=w342) -> (x*y=w344:dbl)
                                n182 = Bundle By Name(cluster=w349, "Drive X Position"=w344) -> (w348:T3)
                                }
                                frame True {
                                }
                                }
                                n183 = local write "Target Position"(w335) -> ()
                              }
                              frame #5 {
                                n184 = Tick Count (ms)() -> (millisecond timer value=w362:u32)
                                n185 = Subtract(x=w362, y=w361) -> (x-y=w364:u32)
                                n186 = Divide(x=w364, y=u32 1000) -> (x/y=w359:dbl)
                                n187 = Build Array (concatenate)(w360, w359) -> (w358:dbl[])
                              }
                              frame #6 {
                                # "update countdown"
                                n188 = Array Size(array=w370) -> (size(s)=w369:i32[])
                                n189 = local read "Mapping Params"() -> (w374:T8)
                                n190 = Index Array(array=w369, index=0) -> (element=w366:i32)
                                n191 = Increment "The data array is not\nyet updated with the\ncurrent run."(x=w366) -> (x+1=w365:i32)
                                n192 = call "Mapping Countdown v10.6.3.vi"("Execution Times (s)"=w371, "Mapping Spectra Settings"=w372, "Ready Steps"=w365, "Mapping Drive Parameters"=w374) -> ("Progress"=→"Progress":i16, "Time String"=w373:string)  [unwired: 6 in]
                                n193 = property on="Measuring" class="Bool (strict)"("BoolText.Text"=w373) -> ()  [unwired: 2 in, 2 out]
                              }
                            }
                            n194 = local read "Start"() -> (w223:bool)
                          }
                        }
                        frame #1 {
                          # "autosave current map"
                          n195 = local read "AutoSave Inc."() -> (w376:i16)
                          n196 = local read "Progress"() -> (w379:u8)
                          n197 = Quotient & Remainder(x=w379, y=w376) -> (floor(x/y)=w381:i16)  [unwired: 1 out]
                          n198 = Quotient & Remainder(x=w382, y=w376) -> (floor(x/y)=w380:i16)  [unwired: 1 out]
                          n199 = Greater?(x=w381, y=w380) -> (0:w378:bool)
                          n200 = Greater Than 0?(x=w376) -> (x > 0?=w377:bool)
                          n201 = And(x=w378, y=w377) -> (x .and. y?=w375:bool)
                          n202 = case shown="True" w375 {
                            tunnel: w385 -> [_ w393]
                            tunnel: w384 -> [_ w392]
                            tunnel: [w386 w389] -> w383
                            tunnel: w382 -> [w386 _]
                            tunnel: w379 -> [_ w389]
                            frame False {
                            }
                            frame True {
                              n203 = local read "Input Parameters"() -> (w406:T1)
                              n204 = global read "Global Variables.vi" "Global iHR Values"() -> (w403:T4)
                              n205 = global read "Global Variables.vi" "Global ITC Values"() -> (w402:T2)
                              n206 = local read "Spectra Params"() -> (w405:T5)
                              n207 = global read "Global Variables.vi" "Global CCD Temperature (C)"() -> (w404:dbl)
                              n208 = Unbundle By Name(w406) -> ("CCD Area"=w407:T6, "CCD Gain"=w409:u16, "CCD ADC"=w408:u16)
                              n209 = Number To Fractional String(number=w389, precision (6)=i16 0) -> (F-format string=w387:string)  [unwired: 2 in]
                              n210 = local read "Mapping Params"() -> (w410:T8)
                              n211 = global read "Global Variables.vi" "Mapping Autosave Folder"() -> (w390:path)
                              n212 = call "Export_mappingFileName v10.5.1.vi"("ITC503 Current Values"=w402, "iHR Current Values"=w403, "Spectra Settings"=w405, "Mapping Parameters"=w410) -> ("Filename"=w397:string)  [unwired: 1 in]
                              n213 = local read "Live Data"() -> (w399:dbl[][])
                              n214 = Unbundle By Name(w410) -> ("Step Size"=w401:dbl)
                              n215 = call "Mapping Merge Real Positions v10.2.1.vi"("Live Data In"=w399, "X in (1D)"=w393, "Y in (1D)"=w392, "Step Size"=w401) -> ("Live Data Out"=w400:dbl[][])  [unwired: 11 in]
                              n216 = Concatenate Strings(w397, "_" ("string"), w387, "pct" ("string")) -> (w394:string)
                              n217 = call "Export_2DtoTxt v10.6.3.vi"("ITC503 Current Values"=w402, "iHR Current Values"=w403, "CCD Temperature"=w404, "CCD Area"=w407, "CCD ADC"=w408, "CCD Gain"=w409, "Auto?"=TRUE, "Export Type"="Mapping", "Spectra Settings"=w405, "Filename"=w394, "Data (2D)"=w400, "Auto Folder"=w390, "Mapping Parameters"=w410) -> ()  [unwired: 6 in, 1 out]
                            }
                          }
                        }
                        frame #2 {
                          # "set new Y and move\nto new position"
                          n218 = Increment(x=w423) -> (x+1=w422:i32)
                          n219 = local read "Start"() -> (w413:bool)
                          n220 = Equal?(x=w421, y=w422) -> (x = y?=w415:bool)
                          n221 = Not(x=w413) -> (.not. x?=w414:bool)
                          n222 = Or(x=w415, y=w414) -> (x .or. y?=w412:bool)
                          n223 = case shown="False" w412 {
                            tunnel: w419 -> [w446 w447]
                            tunnel: [w445 w447] -> w417
                            tunnel: w420 -> [w439 _]
                            frame False {
                              n224 = Unbundle By Name(w446) -> ("Drive Y Position"=w440:dbl)
                              n225 = Add(x=w440, y=w439) -> (x+y=w442:dbl)
                              n226 = Divide(x=w442, y=w439) -> (x/y=w443:dbl)
                              n227 = Round To Nearest(number=w443) -> (nearest integer value=w444:dbl)
                              n228 = Multiply(x=w444, y=w439) -> (x*y=w441:dbl)
                              n229 = Bundle By Name(cluster=w446, "Drive Y Position"=w441) -> (w445:T3)
                            }
                            frame True {
                            }
                          }
                          n230 = local read "Simulate Drive"() -> (w416:bool)
                          n231 = case shown="False" w416 {
                            tunnel: w418 -> [w428 _]
                            tunnel: w417 -> [w427 _]
                            tunnel: w411 -> [w425 _]
                            frame False {
                              n232 = flat-sequence {
                                tunnel: w428 -> [w434]
                                tunnel: w427 -> [w433]
                                tunnel: [w434] -> w429
                                tunnel: w425 -> [w430]
                                tunnel: [w430] -> w424
                                tunnel: [w438] -> w426
                                tunnel: w429 -> [w437]
                                tunnel: w424 -> [w436]
                                frame #0 {
                                n233 = Unbundle By Name(w433) -> ("Drive Y Position"=w432:dbl)
                                n234 = control-ref of="Objective Running"() -> (w435:refnum<vi>)
                                n235 = call "NPC3SG Move Axis To v10.6.2.vi"("Drive Visa Name"=w434, "Running"=w435, "Axis"=1, "Drive Set"=w432, "Calibration File"=w430) -> ()  [unwired: 2 in, 1 out]
                                }
                                frame #1 {
                                n236 = call "NPC3SG Get Positions v10.6.2.vi"("Drive Visa Name"=w437, "Calibration File"=w436) -> ("Drive Current Values"=w438:T3)  [unwired: 5 in]
                                }
                              }
                              n237 = global write "Global Variables.vi" "Global Piezo Position"(w426) -> ()
                              n238 = local write "Current Position"(w426) -> ()
                            }
                            frame True {
                            }
                          }
                          n239 = local write "Target Position"(w417) -> ()
                        }
                      }
                      n240 = local read "Start"() -> (w164:bool)
                    }
                  }
                  frame #2 {
                    # "conclude measurement"
                    n241 = flat-sequence {
                      tunnel: w449 -> [w462]
                      tunnel: w448 -> [w461]
                      tunnel: w450 -> [w467]
                      frame #0 {
                        # "save data"
                        n242 = local read "Input Parameters"() -> (w455:T1)
                        n243 = global read "Global Variables.vi" "Global iHR Values"() -> (w458:T4)
                        n244 = global read "Global Variables.vi" "Global ITC Values"() -> (w459:T2)
                        n245 = local read "Spectra Params"() -> (w456:T5)
                        n246 = global read "Global Variables.vi" "Global CCD Temperature (C)"() -> (w457:dbl)
                        n247 = Unbundle By Name(w455) -> ("CCD Area"=w454:T6, "CCD Gain"=w452:u16, "CCD ADC"=w453:u16)
                        n248 = local read "Mapping Params"() -> (w451:T8)
                        n249 = call "Export_mappingFileName v10.5.1.vi"("ITC503 Current Values"=w459, "iHR Current Values"=w458, "Spectra Settings"=w456, "Mapping Parameters"=w451) -> ("Filename"=w465:string)  [unwired: 1 in]
                        "Filename" <- w465
                        n250 = local read "Live Data"() -> (w464:dbl[][])
                        n251 = Unbundle By Name(w451) -> ("Step Size"=w460:dbl)
                        n252 = call "Mapping Merge Real Positions v10.2.1.vi"("Live Data In"=w464, "X in (1D)"=w462, "Y in (1D)"=w461, "Step Size"=w460) -> ("Live Data Out"=w463:dbl[][])  [unwired: 11 in]
                        "Full Data" <- w463
                        n253 = call "Export_2DtoTxt v10.6.3.vi"("ITC503 Current Values"=w459, "iHR Current Values"=w458, "CCD Temperature"=w457, "CCD Area"=w454, "CCD ADC"=w453, "CCD Gain"=w452, "Export Type"="Mapping", "Spectra Settings"=w456, "Filename"=w465, "Data (2D)"=w463, "Mapping Parameters"=w451) -> ()  [unwired: 8 in, 1 out]
                      }
                      frame #1 {
                        # "reset indicators"
                        n254 = local write "Start"(FALSE ("Start")) -> ()
                        n255 = local write "CCD Current Rep."("0/0" ("CCD3000 Current Rep.")) -> ()
                        n256 = case shown="False" w467 {
                          frame False {
                            n257 = call "Video Toolset Stop.vi"() -> ()  [unwired: 3 in]
                          }
                          frame True {
                          }
                        }
                        n258 = property on="Measuring" class="Bool (strict)"("BoolText.Text"="" ("Boolescher Text.Text")) -> ()  [unwired: 2 in, 2 out]
                        n259 = property on="Measuring" class="Bool (strict)"("Blinking"=FALSE ("Measuring")) -> ()  [unwired: 2 in, 2 out]
                        n260 = global write "Global Variables.vi" "Mapping Running?"(FALSE ("Mapping Running?")) -> ()
                      }
                    }
                  }
                }
              }
            }
          }
          event "Measure Dummy": Value Change {
            n261 = event-data() -> ()  [unwired: 1 in, 5 out]
          }
        }
        n262 = local read "Exit"() -> (w47:bool)
      }
    }
    frame #2 {
      n263 = invoke class="VI Interface Type 0" method="Ctrl Val.Set"(reference=w474, "Control Name"="Exit" ("Elementname"), "Value"=TRUE) -> ()  [unwired: 2 in, 5 out]
      n264 = local read "AutoClose"() -> (w473:bool)
      n265 = flat-sequence {
        tunnel: w473 -> [w477]
        frame #0 {
          # "reset and close"
          n266 = control-ref of="Dieses VI"() -> (w480:refnum<vi>)
          n267 = global write "Global Variables.vi" "Mapping Open?"(FALSE ("Mapping Open?")) -> ()
          n268 = invoke class="VI" method="Default Vals.Reinit All"(reference=w480) -> (reference out=w478:refnum<vi>)  [unwired: 2 in, 2 out]
          n269 = property on="Measuring" class="Bool (strict)"("BoolText.Text"="" ("Boolescher Text.Text")) -> ()  [unwired: 2 in, 2 out]
          n270 = property class="App"() -> ("App.Kind"=w481:T12)  [unwired: 2 in, 2 out]
          n271 = case shown="\"invalid app kind\", Default" w481 {
            tunnel: w478 -> [w483 w485]
            tunnel: w477 -> [_ w484]
            frame "invalid app kind", Default {
              n272 = invoke on="Invoke Node" class="VI" method="FP.Close"(reference=w483) -> ()  [unwired: 2 in, 3 out]
            }
            frame "Development System" {
              n273 = case shown="True" w484 {
                tunnel: w485 -> [_ w486]
                frame False {
                }
                frame True {
                  n274 = invoke on="Invoke Node" class="VI" method="FP.Close"(reference=w486) -> ()  [unwired: 2 in, 3 out]
                }
              }
            }
          }
        }
      }
    }
  }
